vi "UT_EField_DAQ_AnalogIO.get voltage.vi"(0 "i ref in":refnum<vi>, 3 "Timeout":i32=10000, 5 "error in":errorcluster caption="Fehler (Eingang, kein Fehler)") -> (11 "voltage":dbl, 14 "i ref out":refnum<vi>, 17 "timed out":bool, 19 "error out":errorcluster caption="Fehler (Ausgang)")   [LabVIEW 2014, in "UT_EField_DAQ_AnalogIO.lvlib"]
doc: "Contact: Falk Ziegler, eMail: info@lab-coding.de"
uses:
  UT_EField_DAQ_AnalogIO.lvlib
  CS_Core/CSApplicationBaseClasses/PSChannelBase/PSChannelBase.lvlib
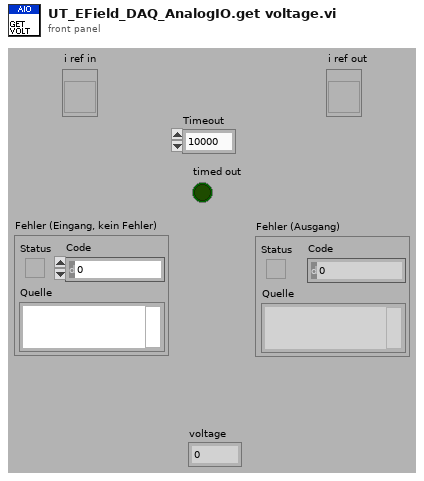
[diagram p1: front panel]
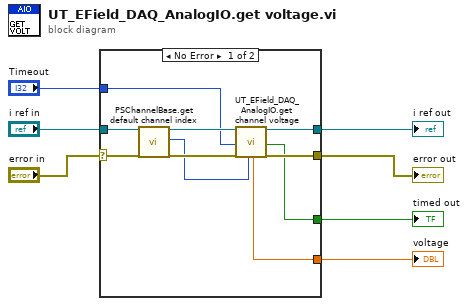
[diagram p0: block diagram]
diagram:
  n1 = case shown="No Error" "error in" {
    selector: "error in" -> [w16 w18]
    tunnel: "i ref in" -> [w17 w19]
    tunnel: [w9 w19] -> w5
    tunnel: "Timeout" -> [w13 _]
    tunnel: [w10 w18] -> w3
    tunnel: [w11 _] -> w2
    tunnel: [w8 _] -> w1
    frame No Error {
      n2 = call "PSChannelBase.get default channel index.vi"("i ref in"=w17, "error in (no error)"=w16) -> ("i ref out"=w15:refnum<vi>, "defaultChannelIndex"=w12:i32, "error out"=w14:errorcluster)  [unwired: 15 in]
      n3 = call "UT_EField_DAQ_AnalogIO.get channel voltage.vi"("i ref in"=w15, "Timeout"=w13, "error in"=w14, "channel_index"=w12) -> ("voltage"=w11:dbl, "i ref out"=w9:refnum<vi>, "timed out"=w8:bool, "error out"=w10:errorcluster)  [unwired: 12 in]
    }
    frame Error {
    }
  }
  "error out" <- w3
  "timed out" <- w1
  "i ref out" <- w5
  "voltage" <- w2
